vi "setFPGAReference.vi"(10 "FPGAReference":refnum<k20>, 11 "MyHealthAndStatusReadFIFO in":refnum<class "MyHealthAndStatusReadFIFO.lvclass">) -> (3 "MyHealthAndStatusReadFIFO out":refnum<class "MyHealthAndStatusReadFIFO.lvclass">)   [LabVIEW 2016, in "MyHealthAndStatusReadFIFO.lvclass"]
uses:
  MyHealthAndStatusReadFIFO.lvclass
  MyHealthAndStatusReadFIFO.lvclass/MyHealthAndStatusReadFIFO.ctl
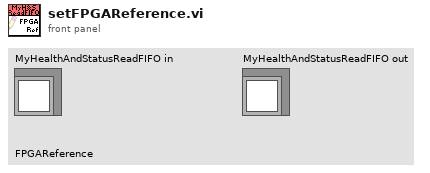
[diagram p1: front panel]
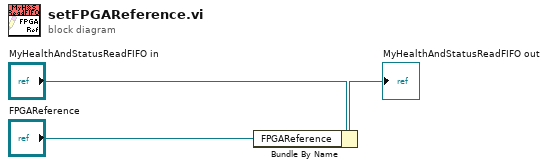
[diagram p0: block diagram]
diagram:
  n1 = Bundle By Name(cluster="MyHealthAndStatusReadFIFO in", "FPGAReference"="FPGAReference") -> (→"MyHealthAndStatusReadFIFO out":refnum<class "MyHealthAndStatusReadFIFO.lvclass">)
